vi "Init.vi"(8 "error in (no error)":errorcluster, 10 "Index":i32, 11 "Group":refnum<class "StringGroup.lvclass">) -> (0 "error out":errorcluster, 3 "StringChannel out":refnum<class "StringChannel.lvclass">)   [LabVIEW 2020, in "Vecto.lvlib" / "StringChannel.lvclass"]
uses:
  StringChannel.lvclass
  StringGroup/StringGroup.lvclass
  StringChannel.lvclass/StringChannel.ctl
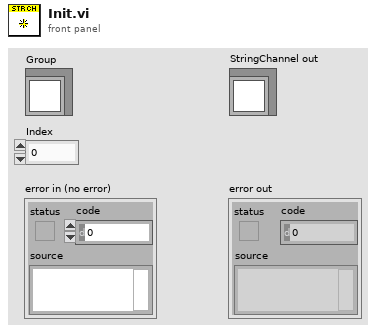
[diagram p1: front panel]
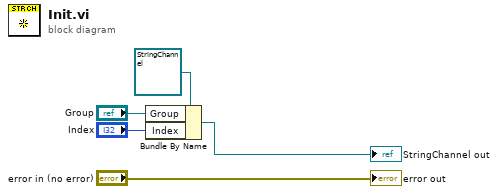
[diagram p0: block diagram]
diagram:
  n1 = Bundle By Name(cluster=refnum<class "StringChannel.lvclass"> refnum ("StringChannel in"), "Group"="Group", "Index"="Index") -> (→"StringChannel out":refnum<class "StringChannel.lvclass">)
  "error out" <- "error in (no error)"
